vi "Update Operating Mode.vi"(10 "UTP IO Session in":T1, 11 "Sequence Context In":refnum<k7>) -> ()   [LabVIEW 2023]
uses:
  <vilib>/Noffz/UTP IO/UTP IO Library/Typedefs/Session Handle.ctl
  <vilib>/Noffz/UTP IO/UTP IO Library/UTP IO Pool Session.lvclass
  <vilib>/Noffz/UTP IO/UTP IO Library/methods/poly/plc/Read PLC Variable (I16).vi
  <vilib>/addons/TestStand/_TSUtility.llb/TestStand - Set Property Value (Number {Signed 16-bit Integer}).vi
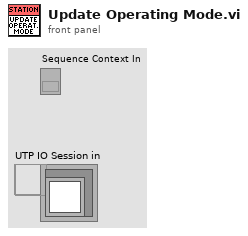
[diagram p1: front panel]
types:
  T1 = typedef "UTP IO Library.lvlib/UTP IO Pool Session.lvclass/Session Handle.ctl" = refnum<data-value>
  T2 = typedef "TestStand - Status Monitor.ctl" = cluster{"Sequence Context":refnum<k7>, "Execution":refnum<k7>, "Termination Monitor":refnum<k7>}
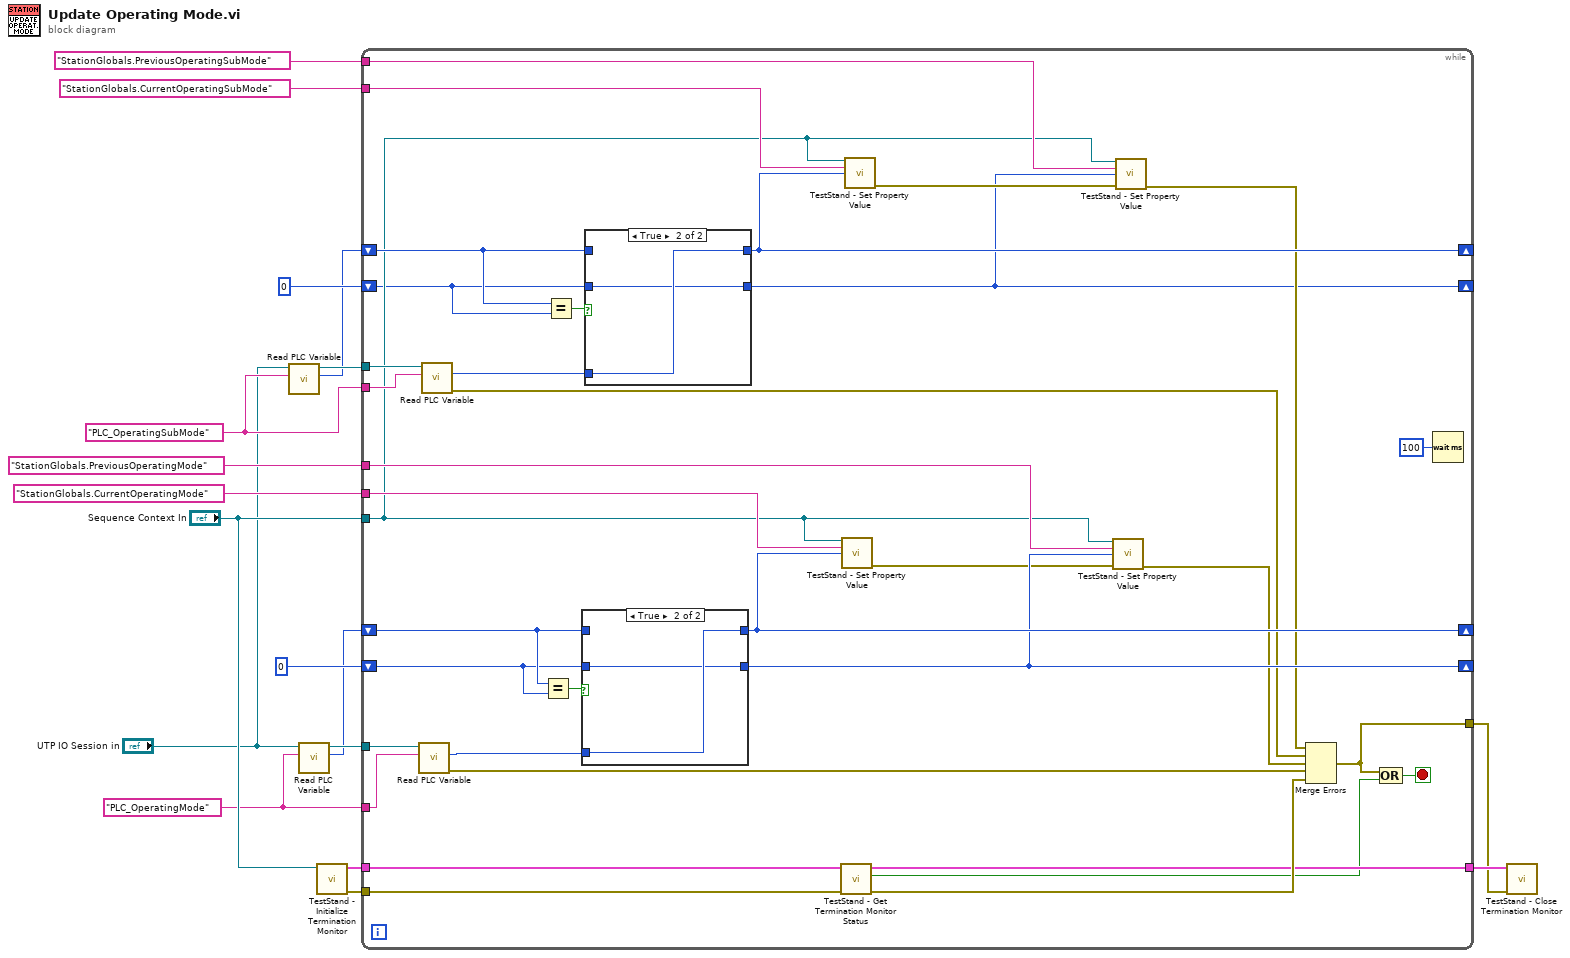
[diagram p0: block diagram]
diagram:
  w6 = "PLC_OperatingSubMode" ("variable name")
  w2 = "PLC_OperatingMode" ("variable name")
  n1 = call-poly <vilib>:"Read PLC Variable.vi"("variable name"=w6, "UTP IO Session in"="UTP IO Session in") -> ("value"=w5:i16, "UTP IO Session out"=w7:T1)  [unwired: 7 in, 1 out]
  n2 = call-poly <vilib>:"Read PLC Variable.vi"("variable name"=w2, "UTP IO Session in"="UTP IO Session in") -> ("value"=w1:i16, "UTP IO Session out"=w3:T1)  [unwired: 7 in, 1 out]
  n3 = call <vilib>:"TestStand - Initialize Termination Monitor.vi"("Sequence Context In"="Sequence Context In") -> ("error out"=w16:errorcluster, "Status Monitor Out"=w15:T2)  [unwired: 9 in]
  n4 = while {
    tunnel: w2 -> [w37]
    shift-right: [w50] -> _
    shift-left: w1 -> [w52]
    shift-right: [w49] -> _
    shift-left: i16 0 ("value") -> [w20]
    tunnel: "Sequence Context In" -> [w24]
    tunnel: w16 -> [w47]
    tunnel: w15 -> [w46]
    tunnel: [w43] -> w14
    tunnel: [w41] -> w13
    tunnel: "StationGlobals.CurrentOperatingMode" ("Lookup String") -> [w39]
    tunnel: "StationGlobals.PreviousOperatingMode" ("Lookup String") -> [w38]
    tunnel: w7 -> [w33]
    tunnel: w6 -> [w34]
    shift-right: [w29] -> _
    shift-left: w5 -> [w28]
    shift-right: [w22] -> _
    shift-left: i16 0 ("value") -> [w23]
    tunnel: "StationGlobals.CurrentOperatingSubMode" ("Lookup String") -> [w31]
    tunnel: "StationGlobals.PreviousOperatingSubMode" ("Lookup String") -> [w32]
    tunnel: w3 -> [w21]
    stop <- w42 stop-if-true
    n5 = call-poly <vilib>:"Read PLC Variable.vi"("variable name"=w37, "UTP IO Session in"=w21) -> ("error out"=w36:errorcluster, "value"=w19:i16)  [unwired: 7 in, 1 out]
    n6 = call-poly <vilib>:"Read PLC Variable.vi"("variable name"=w34, "UTP IO Session in"=w33) -> ("error out"=w26:errorcluster, "value"=w35:i16)  [unwired: 7 in, 1 out]
    n7 = Equal?(x=w52, y=w20) -> (x = y?=w53:bool)
    n8 = Equal?(x=w28, y=w23) -> (x = y?=w27:bool)
    n9 = case shown="True" w53 {
      tunnel: [w57 w59] -> w50
      tunnel: [w57 w58] -> w49
      tunnel: w20 -> [_ w58]
      tunnel: w52 -> [_ _]
      tunnel: w19 -> [w57 w59]
      frame False {
      }
      frame True {
      }
    }
    n10 = case shown="True" w27 {
      tunnel: w35 -> [w54 w56]
      tunnel: [w54 w56] -> w29
      tunnel: w23 -> [_ w55]
      tunnel: w28 -> [_ _]
      tunnel: [w54 w55] -> w22
      frame False {
      }
      frame True {
      }
    }
    n11 = call <vilib>:"TestStand - Get Termination Monitor Status.vi"("error in (no error)"=w47, "Status Monitor In"=w46) -> ("error out"=w44:errorcluster, "Terminating or Aborting"=w40:bool, "Status Monitor Out"=w43:T2)  [unwired: 7 in]
    n12 = call-poly <vilib>:"TestStand - Set Property Value.vi"("Sequence Context In"=w24, "Lookup String"=w39, "New Value"=w50) -> ("error out"=w48:errorcluster)  [unwired: 11 in, 1 out]
    n13 = call-poly <vilib>:"TestStand - Set Property Value.vi"("Sequence Context In"=w24, "Lookup String"=w31, "New Value"=w29) -> ("error out"=w30:errorcluster)  [unwired: 11 in, 1 out]
    n14 = call-poly <vilib>:"TestStand - Set Property Value.vi"("Sequence Context In"=w24, "Lookup String"=w38, "New Value"=w49, "error in (no error)"=w48) -> ("error out"=w45:errorcluster)  [unwired: 10 in, 1 out]
    n15 = call-poly <vilib>:"TestStand - Set Property Value.vi"("Sequence Context In"=w24, "Lookup String"=w32, "New Value"=w22, "error in (no error)"=w30) -> ("error out"=w25:errorcluster)  [unwired: 10 in, 1 out]
    n16 = Merge Errors(w25, w26, w45, w36, w44) -> (w41:errorcluster)
    n17 = Compound Arithmetic op=OR(w41, w40) -> (w42:bool)
    n18 = Wait (ms)(milliseconds to wait=u32 100) -> ()  [unwired: 1 out]
  }
  n19 = call <vilib>:"TestStand - Close Termination Monitor.vi"("error in (no error)"=w13, "Status Monitor In"=w14) -> ()  [unwired: 9 in, 1 out]
